vi "configure.vi"(8 "error in (no error)":errorcluster, 11 "TrajectoryRK110428Fiber in":refnum<class "TrajectoryRK110428Fiber_Spiral.lvclass">) -> (0 "error out":errorcluster, 3 "TrajectoryRK110428Fiber out":refnum<class "TrajectoryRK110428Fiber_Spiral.lvclass">)   [LabVIEW 2010, in "TrajectoryRK110428Fiber_Spiral.lvclass"]
doc: "The dynamic dispatch version of this VI loads and displays the configuration file associated with the plug-in object. The user modify and save the configuration data."
uses:
  TrajectoryRK110428Fiber_Spiral.lvclass
  common/xcontrols/XComponentSpecification/XComponentSpecification/XComponentSpecification.xctl
  TrajectoryRK110428Fiber_Spiral.lvclass/TrajectoryRK110428Fiber_Spiral.ctl
  common/classes/GenericComponent/GenericComponent/GenericComponent.lvclass
panel:
  in  "Cancel":bool
  in  "Save":bool
  in  "Tab Control":enum32{"Description", "FPGA Wrapper"}(tab)
  in  "FPGAWrapper spec":T1(xcontrol)
  out "Configuration name":string
  # "Configure TrajectoryRK110428Fiber_Spiral"
  # "The TrajectoryRK110428Fiber_Spiral components controls the fiber scanner spiral trajectory for the FPGA.\n\nThe FPGA controls the DAC in the HIFO box version2 that synthesizes the spiral waveform for the piezo fiber scanner."
  # "FPGA Wrapper"
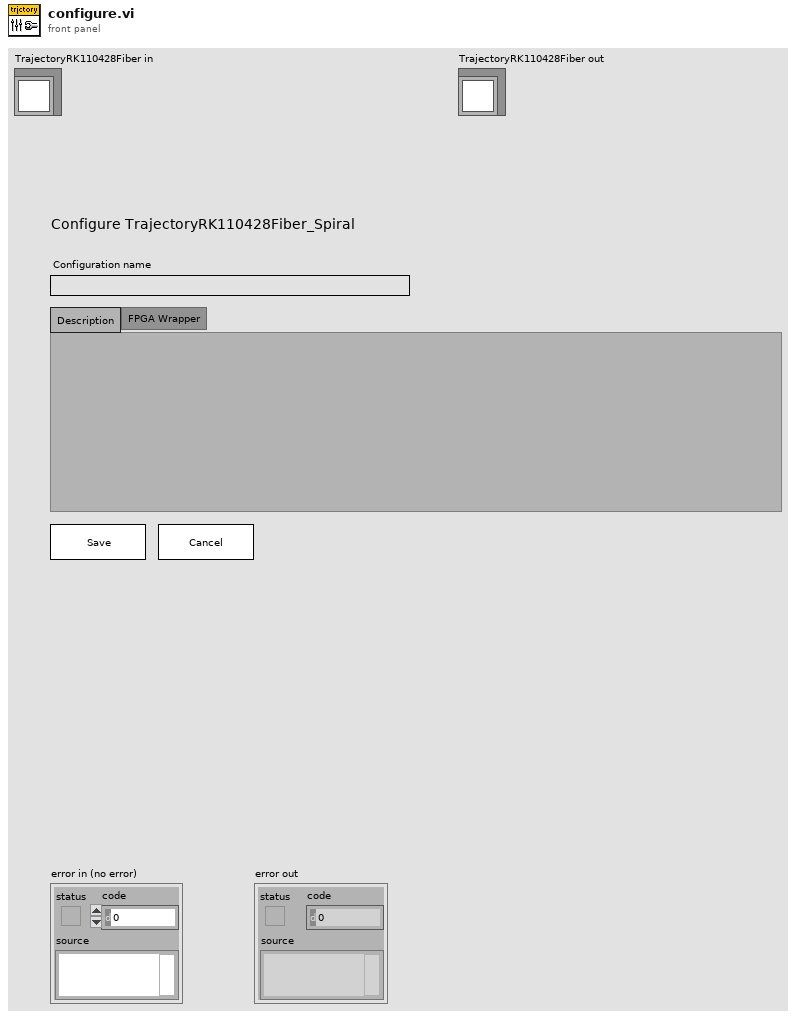
[diagram p1: front panel]
types:
  T1 = cluster{"class path":string, "configuration":string, "label":string, "settings name":string}
  T2 = typedef "plugin_specification.ctl" = cluster{"class path":string, "configuration":string, "label":string, "settings name":string}
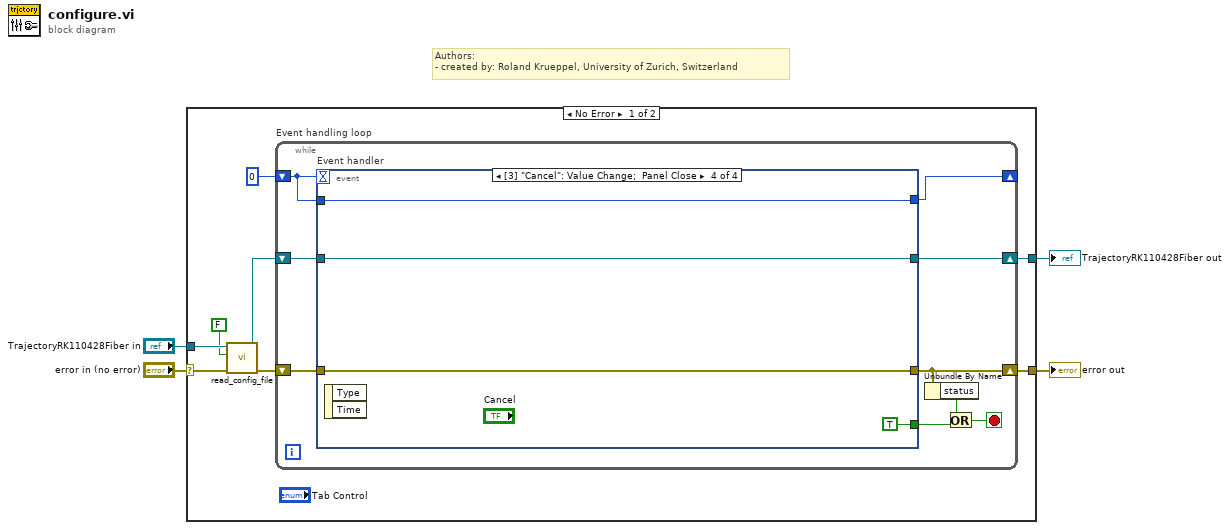
[diagram p0: block diagram]
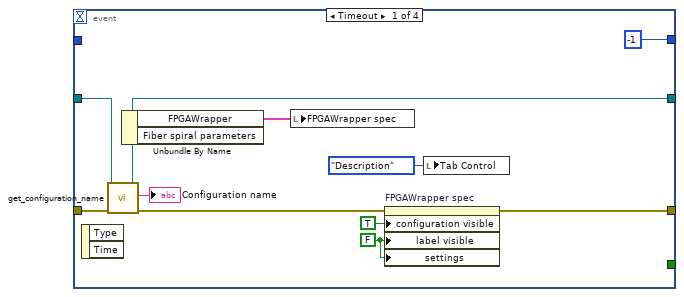
[diagram p2: hidden frame]
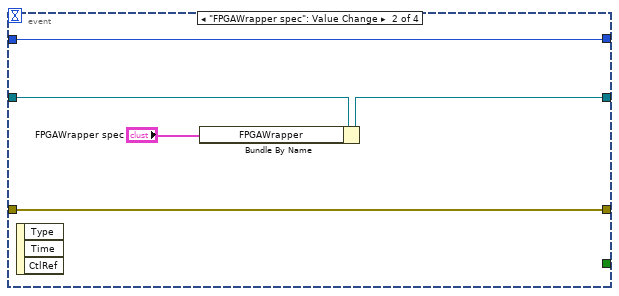
[diagram p3: hidden frame]
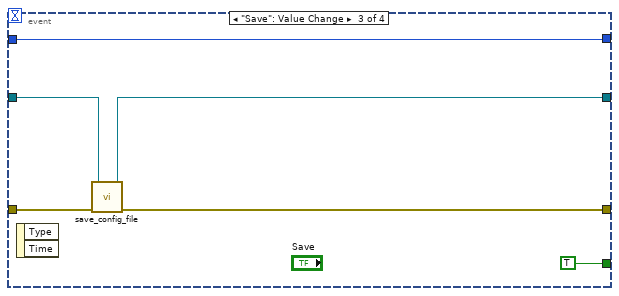
[diagram p4: hidden frame]
diagram:
  # "Authors: \n- created by: Roland Krueppel, University of Zurich, Switzerland"
  n1 = case shown="No Error" "error in (no error)" {
    selector: "error in (no error)" -> [w12 w48]
    tunnel: "TrajectoryRK110428Fiber in" -> [w11 w49]
    tunnel: [w6 w48] -> w2
    tunnel: [w5 w49] -> w1
    frame No Error {
      n2 = call-dynamic "read_config_file.vi"("error in (no error)"=w12, "force load?"=FALSE, "GenericPlugin in"=w11) -> ("error out"=w8:errorcluster, "GenericPlugin out"=w9:refnum<class "TrajectoryRK110428Fiber_Spiral.lvclass">)  [unwired: 7 in]
      n3 = while "Event handling loop" {
        shift-right: [w18] -> w5
        shift-left: w9 -> [w21]
        shift-right: [w16] -> w6
        shift-left: w8 -> [w20]
        shift-right: [w17] -> _
        shift-left: 0 -> [w19]
        stop <- w15 stop-if-true
        n4 = event "Event handler" shown="[3] \"Cancel\": Value Change;  Panel Close" {
          selector: _ -> [_ _ _ _]
          dyn-events: _ -> [_ _ _ _]
          timeout: w19 -> [_ _ _ _]
          tunnel: w21 -> [w32 w35 w41 w47]
          tunnel: w20 -> [w31 w36 w43 w46]
          tunnel: w19 -> [_ w37 w38 w44]
          tunnel: [w23 w34 w40 w47] -> w18
          tunnel: [w25 w36 w42 w46] -> w16
          tunnel: [-1 w37 w38 w44] -> w17
          tunnel: [_ _ TRUE TRUE] -> w14
          event Timeout {
            w26 = FALSE ("label visible")
            n5 = event-data() -> ()  [unwired: 1 in, 2 out]
            n6 = call "get_configuration_name.vi"("error in (no error)"=w31, "GenericPlugin.lvclass in"=w32) -> ("error out"=w28:errorcluster, "configuration name"=→"Configuration name":string, "GenericPlugin.lvclass out"=w23:refnum<class "TrajectoryRK110428Fiber_Spiral.lvclass">)  [unwired: 7 in]
            n7 = Unbundle By Name(w23) -> ("FPGAWrapper"=w24:T2)  [unwired: 1 out]
            n8 = local write "FPGAWrapper spec"(w24) -> ()
            n9 = property on="FPGAWrapper spec" class="XComponentSpecification (strict"(error in=w28, "configuration visible"=TRUE, "label visible"=w26, "settings"=w26) -> (error out=w25:errorcluster)  [unwired: 1 in, 1 out]
            n10 = local write "Tab Control"(enum32{"Description", "FPGA Wrapper"}."Description" ("Tab Control")) -> ()
          }
          event "FPGAWrapper spec": Value Change {
            n11 = event-data() -> ()  [unwired: 1 in, 3 out]
            n12 = Bundle By Name(cluster=w35, "FPGAWrapper"="FPGAWrapper spec") -> (w34:refnum<class "TrajectoryRK110428Fiber_Spiral.lvclass">)
          }
          event "Save": Value Change {
            n13 = event-data() -> ()  [unwired: 1 in, 2 out]
            n14 = call-dynamic "save_config_file.vi"("error in (no error)"=w43, "GenericPlugin in"=w41) -> ("error out"=w42:errorcluster, "GenericPlugin out"=w40:refnum<class "TrajectoryRK110428Fiber_Spiral.lvclass">)  [unwired: 8 in]
          }
          event "Cancel": Value Change; Panel Close {
            n15 = event-data() -> ()  [unwired: 1 in, 2 out]
          }
        }
        n16 = Unbundle By Name(w16) -> ("status"=w13:bool)
        n17 = Or(x=w13, y=w14) -> (x .or. y?=w15:bool)
      }
    }
    frame Error {
    }
  }
  "error out" <- w2
  "TrajectoryRK110428Fiber out" <- w1
